vi "Warning Messages.vi"(11 "Powerdown?":bool) -> (3 "Warning Messages":string[](array[string]))   [LabVIEW 2024, in "devicePowerSequencerCoreLogic.lvlib"]
uses:
  devicePowerSequencerCoreLogic.lvlib
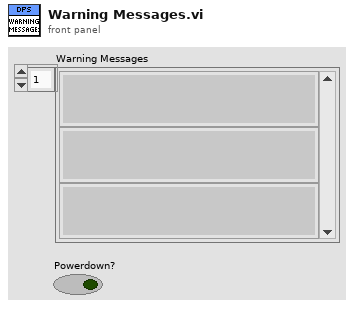
[diagram p1: front panel]
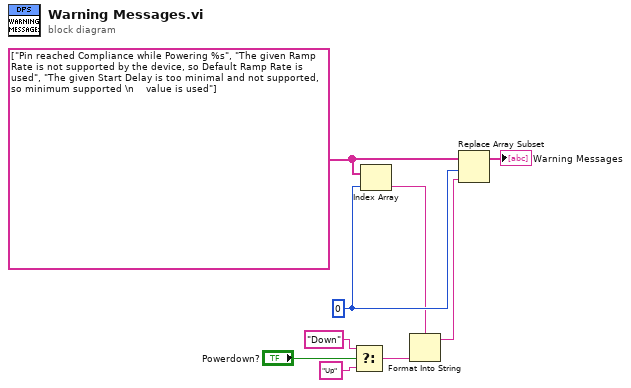
[diagram p0: block diagram]
diagram:
  w2 = 0 ("index")
  w3 = string[] ["Pin reached Compliance while Powering %s", "The given Ramp Rate is not supported by the device, so Default Ramp Rate is used", "The given Start Delay is too minimal and not supported, so minimum supported \n    value is used"]
  n1 = Select(t="Down", s="Powerdown?", f="Up") -> (s? t:f=w7:string)
  n2 = Index Array(array=w3, index=w2) -> (element=w1:string)
  n3 = Format Into String(format string=w1, w7) -> (resulting string=w8:string)  [unwired: 2 in, 1 out]
  n4 = Replace Array Subset(array=w3, new element=w8, index=w2) -> (→"Warning Messages":string[])
